vi "Check if Queue is Registered.vi"(8 "error in (no error)":errorcluster, 11 "name (unnamed)":string) -> (0 "error out":errorcluster, 1 "Registered?":bool, 3 "Registered Queue":refnum<queue>)   [LabVIEW 2020]
doc: "This VI checks to see if a queue is in the Queue Registry.\n\nIf the queue is in the registry, Registered? is true and the queue is returned. If it is not, Registred is false and an empty queue is returned."
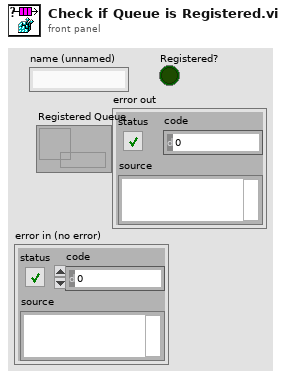
[diagram p1: front panel]
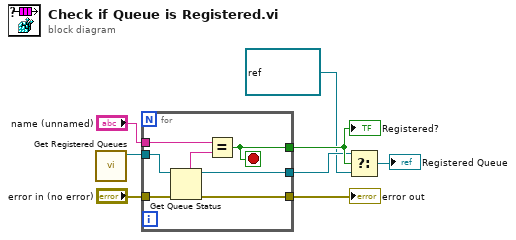
[diagram p0: block diagram]
diagram:
  n1 = call "Get Registered Queues.vi"() -> ("Queue Registry"=w7:refnum<notifier>)  [unwired: 9 in, 2 out]
  n2 = for {
    tunnel: w7 -> [w15]
    tunnel: "name (unnamed)" -> [w14]
    tunnel: [w12] -> w3
    tunnel: [w11] -> w4
    tunnel: "error in (no error)" -> [w10]
    tunnel: [w9] -> w5
    stop <- w11 stop-if-true
    n3 = Get Queue Status(queue=w15, error in (no error)=w10) -> (queue out=w12:refnum<queue>, queue name=w13:string, error out=w9:errorcluster)  [unwired: 1 in, 5 out]
    n4 = Equal?(x=w14, y=w13) -> (x = y?=w11:bool)
  }
  "Registered?" <- w4
  "error out" <- w5
  n5 = Select(t=w3, s=w4, f=refnum<queue> refnum) -> (s? t:f=→"Registered Queue":refnum<queue>)
